vi "mes~Login Dialog.vi"(8 "错误输入（无错误）":errorcluster) -> (0 "错误常量":errorcluster, 2 "Success?":bool)   [LabVIEW 2020]
uses:
  <vilib>/Utility/miscctls.llb/LVPointTypeDef.ctl
  Global.vi
panel:
  in  "登录":bool
  in  "Password":string caption="密   码:"
  in  "UserName":string caption="用户名:"
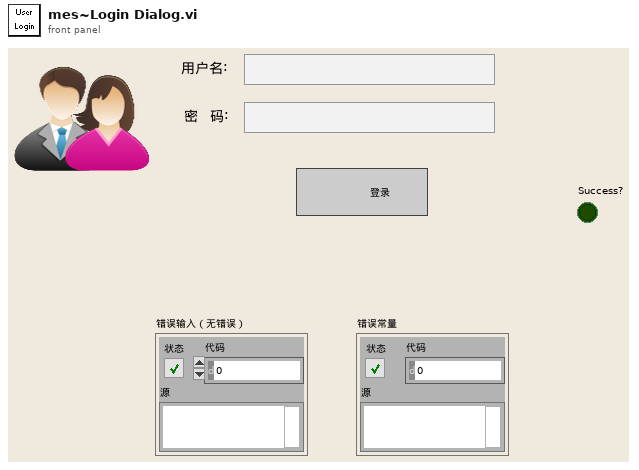
[diagram p1: front panel]
types:
  T1 = typedef "LVPointTypeDef.ctl" = cluster{"Horizontal":i16, "Vertical":i16}
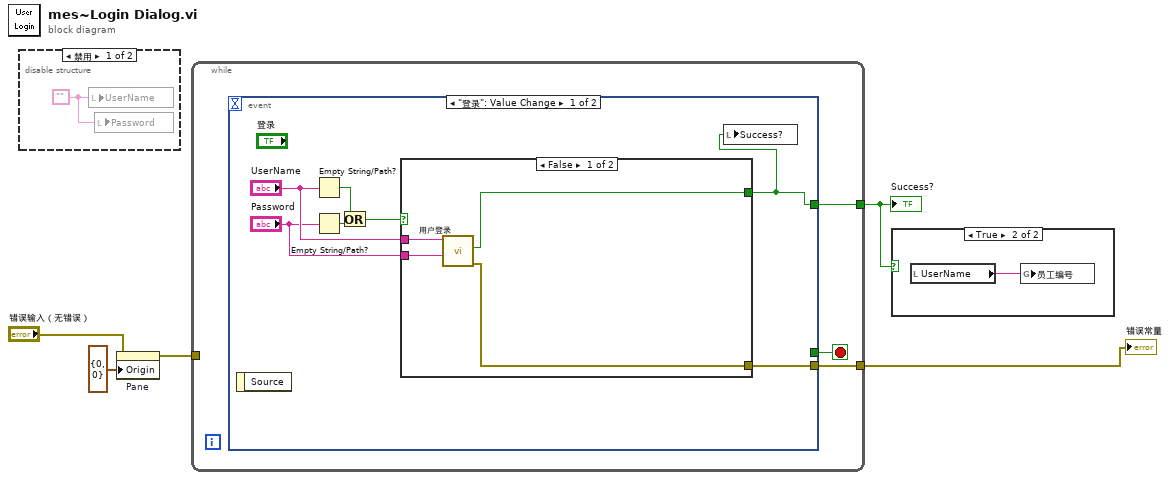
[diagram p0: block diagram]
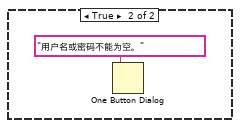
[diagram p4: hidden frame]
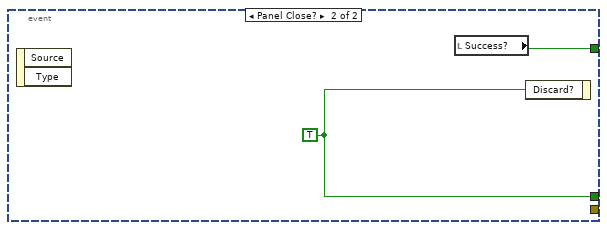
[diagram p5: hidden frame]
diagram:
  n1 = disable-structure shown="禁用" {
    frame Disabled {
      w6 = ""
      n2 = local write "UserName"(w6) -> ()
      n3 = local write "Password"(w6) -> ()
    }
    frame Enabled {
    }
  }
  n4 = property on="Pane" class="Pane"(error in="错误输入（无错误）", "Origin"=T1 {"Horizontal"=0, "Vertical"=0}) -> (error out=w4:errorcluster)  [unwired: 1 in, 1 out]
  n5 = while {
    tunnel: [w8] -> w3
    tunnel: w4 -> [_]
    tunnel: [w7] -> w1
    stop <- w9 stop-if-true
    n6 = event shown="[0] \"登录\": Value Change" {
      selector: _ -> [_ _]
      dyn-events: _ -> [_ _]
      timeout: _ -> [_ _]
      tunnel: [_ w23] -> w9
      tunnel: [w11 w22] -> w8
      tunnel: [w10 _] -> w7
      event "登录": Value Change {
        n7 = event-data() -> ()  [unwired: 1 in, 1 out]
        n8 = Empty String/Path?(string/path="UserName") -> (empty?=w15:bool)
        n9 = Empty String/Path?(string/path="Password") -> (empty?=w16:bool)
        n10 = Or(x=w15, y=w16) -> (x .or. y?=w14:bool)
        n11 = case shown="False" w14 {
          tunnel: "UserName" -> [w20 _]
          tunnel: "Password" -> [w19 _]
          tunnel: [w18 _] -> w11
          tunnel: [w17 _] -> w10
          frame False {
            n12 = call "用户登录.vi"("Password"=w19, "UserName"=w20) -> ("error out"=w17:errorcluster, "登录成功"=w18:bool)  [unwired: 7 in, 1 out]
          }
          frame True {
            n13 = One Button Dialog(message="用户名或密码不能为空。") -> ()  [unwired: 1 in, 1 out]
          }
        }
        n14 = local write "Success?"(w11) -> ()
      }
      event Panel Close? {
        w23 = TRUE
        n15 = event-data() -> ()  [unwired: 1 in, 2 out]
        n16 = local read "Success?"() -> (w22:bool)
        n17 = event-data("Discard?"=w23) -> ()  [unwired: 1 in, 1 out]
      }
    }
  }
  "Success?" <- w3
  "错误常量" <- w1
  n18 = case shown="True" w3 {
    frame False {
    }
    frame True {
      n19 = local read "UserName"() -> (w24:string)
      n20 = global write "Global.vi" "员工编号"(w24) -> ()
    }
  }
